vi "Auto settings.vi"(8 "error in (no error)":errorcluster, 10 "Array":dbl[](array[numeric]), 11 "Assembly Tray in":refnum<class "Assembly Tray.lvclass">) -> (0 "error out":errorcluster, 3 "Assembly Tray out":refnum<class "Assembly Tray.lvclass">)   [LabVIEW 2021, in "Assembly Tray.lvclass"]
uses:
  Assembly Tray.lvclass
  C:/Users/HEP/Documents/GitHub/UCSB-Gantry-HEP/Classes/Workspace/Fixture.lvclass
  Assembly Tray.lvclass/Assembly Tray.ctl
  Fixture.lvclass/Fixture.ctl
  Write Gantry Region.vi
  Write Position.vi
  Write Fixture ID.vi
panel:
  out "Component thickness out":dbl
  in  "Component Thickness":dbl=1.46685 format="%#_13g"
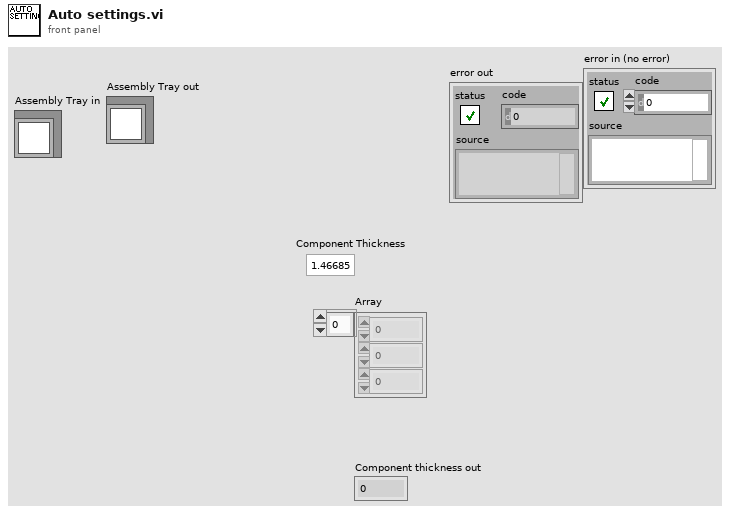
[diagram p1: front panel]
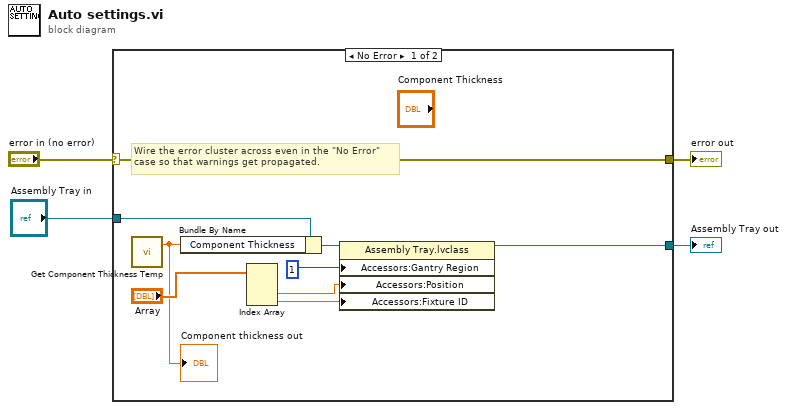
[diagram p0: block diagram]
diagram:
  n1 = case shown="No Error" "error in (no error)" {
    selector: "error in (no error)" -> [w13 w15]
    tunnel: [w13 w15] -> w3
    tunnel: [w12 w14] -> w1
    tunnel: "Assembly Tray in" -> [w11 w14]
    frame No Error {
      # "Wire the error cluster across even in the \"No Error\"\ncase so that warnings get propagated."
      n2 = call "Get Component Thickness Temp.vi"() -> ("Component Thickness out"=w6:dbl)  [unwired: 5 in]
      "Component thickness out" <- w6
      n3 = Bundle By Name(cluster=w11, "Component Thickness"=w6) -> (w10:refnum<class "Assembly Tray.lvclass">)
      n4 = Index Array(array="Array") -> (element #2=w8:dbl, element #3=w7:dbl)  [unwired: 3 in, 1 out]
      n5 = property class="Assembly Tray.lvclass"(reference=w10, "Accessors:Gantry Region"=1 ("Gantry Region"), "Accessors:Position"=w8, "Accessors:Fixture ID"=w7) -> (reference out=w12:refnum<class "Assembly Tray.lvclass">)  [unwired: 1 in, 1 out]
    }
    frame Error {
    }
  }
  "error out" <- w3
  "Assembly Tray out" <- w1
